vi "RichToFlatnixnet_grpc_DbGetDatabaseListSizesResponse.vi"(5 "OutputClusterType":T1, 11 "InputCluster":T2) -> (3 "OutputCluster":T1)   [LabVIEW 2025, in "xnet-grpc_client.lvlib"]
uses:
  nixnet_grpc_DbGetDatabaseListSizesResponse.ctl
  nixnet_grpc_DbGetDatabaseListSizesResponse_Flat.ctl
  xnet-grpc_client.lvlib
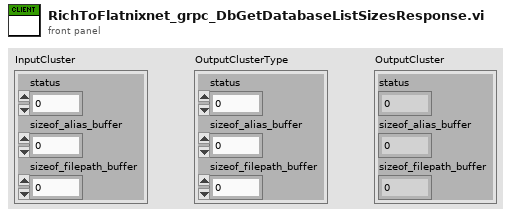
[diagram p1: front panel]
types:
  T1 = typedef "xnet-grpc_client.lvlib/nixnet_grpc_DbGetDatabaseListSizesResponse_Flat.ctl" = cluster{"status":i32, "sizeof_alias_buffer":u32, "sizeof_filepath_buffer":u32}
  T2 = typedef "xnet-grpc_client.lvlib/nixnet_grpc_DbGetDatabaseListSizesResponse.ctl" = cluster{"status":i32, "sizeof_alias_buffer":u32, "sizeof_filepath_buffer":u32}
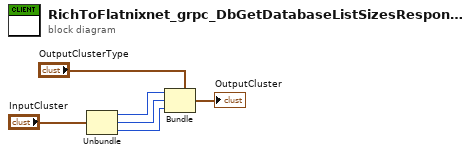
[diagram p0: block diagram]
diagram:
  n1 = Unbundle "Unbundle"("InputCluster") -> ("status"=w3:i32, "sizeof_alias_buffer"=w2:u32, "sizeof_filepath_buffer"=w1:u32)
  n2 = Bundle "Bundle"(cluster="OutputClusterType", "status"=w3, "sizeof_alias_buffer"=w2, "sizeof_filepath_buffer"=w1) -> (→"OutputCluster":T1)
